vi "ScriptCopyPasteAll.vi"(8 "error in (no error)":errorcluster, 11 "VI in":refnum<vi>) -> (0 "error out":errorcluster, 3 "VI out":refnum<vi>)   [LabVIEW 2014]
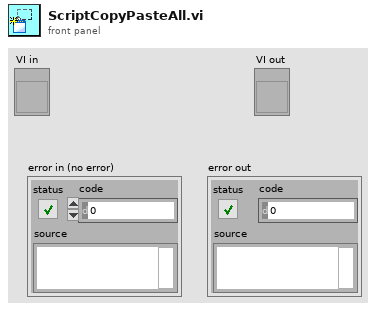
[diagram p1: front panel]
types:
  T1 = typedef "LVPositionTypeDef.ctl" = cluster{"Left":i32, "Top":i32}
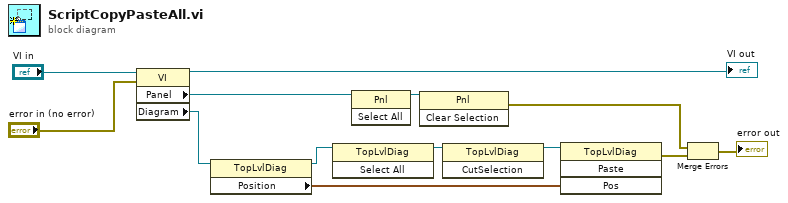
[diagram p0: block diagram]
diagram:
  n1 = property class="VI"(reference="VI in", error in="error in (no error)") -> (reference out=→"VI out":refnum<vi>, "Panel"=w13:refnum<vi>, "Diagram"=w3:refnum<vi>)  [unwired: 1 out]
  n2 = property class="TopLvlDiag"(reference=w3) -> (reference out=w1:refnum<vi>, "Position"=w2:T1)  [unwired: 1 in, 1 out]
  n3 = invoke class="TopLvlDiag" method="Select All"(reference=w1) -> (reference out=w12:refnum<vi>)  [unwired: 2 in, 2 out]
  n4 = invoke class="Pnl" method="Select All"(reference=w13) -> (reference out=w11:refnum<vi>)  [unwired: 2 in, 2 out]
  n5 = invoke class="Pnl" method="Clear Selection"(reference=w11) -> (error out=w5:errorcluster)  [unwired: 2 in, 2 out]
  n6 = invoke class="TopLvlDiag" method="CutSelection"(reference=w12) -> (reference out=w7:refnum<vi>)  [unwired: 2 in, 2 out]
  n7 = invoke class="TopLvlDiag" method="Paste"(reference=w7, "Pos"=w2) -> (error out=w6:errorcluster)  [unwired: 2 in, 3 out]
  n8 = Merge Errors(w5, w6) -> (→"error out":errorcluster)
